vi "Get Boolean Trigger.vi"(7 "Trigger Direction":T1, 8 "error in (no error)":errorcluster, 11 "Item Ref in":T3 format="%.0x") -> (0 "error out":errorcluster, 2 "Boolean Trigger":T2, 3 "Item Ref out":T3 format="%.0x")   [LabVIEW 2012, in "Waveform Data Logger Shared.lvlib"]
uses:
  Waveform Data Logger Shared.lvlib
  <vilib>/NI Veristand/Custom Device API/Custom Device Item Ref.ctl
  Types/Boolean Trigger.ctl
  Types/Trigger Direction.ctl
  Globals/Property Strings.vi
  <vilib>/NI Veristand/Custom Device API/Get Item Property (Double).vi
  <vilib>/NI Veristand/Custom Device API/Get Item Property (U16).vi
  <vilib>/NI VeriStand/Custom Device API/Custom Device API.lvlib
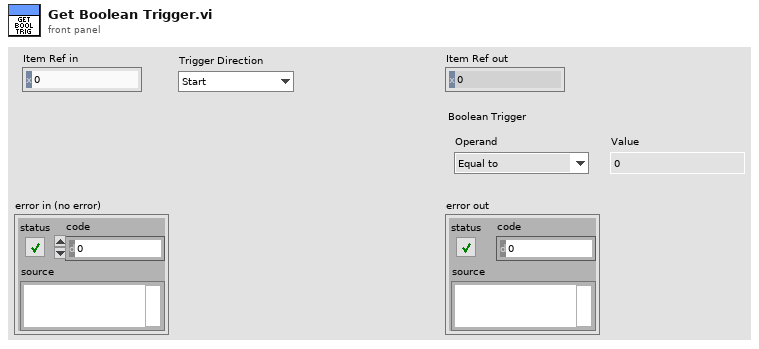
[diagram p1: front panel]
types:
  T1 = typedef "Waveform Data Logger Shared.lvlib/Trigger Direction.ctl" = enum16{"Start", "Stop"}
  T2 = typedef "Waveform Data Logger Shared.lvlib/Boolean Trigger.ctl" = cluster{"Value":dbl, "Operand":enum16{"Equal to", "Not equal to", "Less than", "Less than or equal", "Greater than", "Greater than or equal"}}
  T3 = typedef "Custom Device API.lvlib/Custom Device Item Ref.ctl" = u64
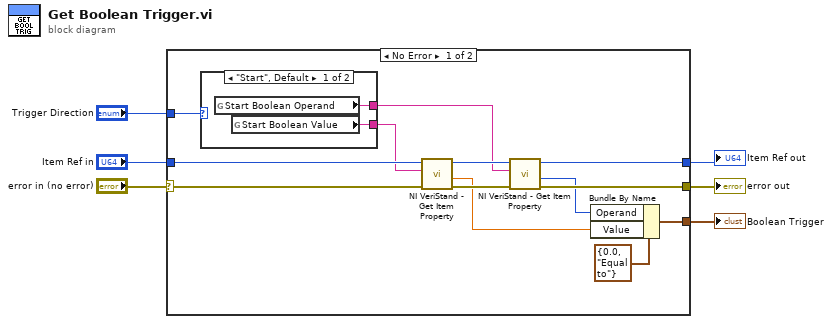
[diagram p0: block diagram]
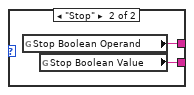
[diagram p2: hidden frame]
diagram:
  n1 = case shown="No Error" "error in (no error)" {
    selector: "error in (no error)" -> [w16 w24]
    tunnel: [w14 w25] -> w6
    tunnel: [w11 w24] -> w5
    tunnel: "Item Ref in" -> [w17 w25]
    tunnel: "Trigger Direction" -> [w19 _]
    tunnel: [w7 _] -> w1
    frame No Error {
      n2 = case shown="\"Start\", Default" w19 {
        tunnel: [w21 w23] -> w10
        tunnel: [w20 w22] -> w15
        frame "Start", Default {
          n3 = global read "Property Strings.vi" "Start Boolean Operand"() -> (w21:string)
          n4 = global read "Property Strings.vi" "Start Boolean Value"() -> (w20:string)
        }
        frame "Stop" {
          n5 = global read "Property Strings.vi" "Stop Boolean Operand"() -> (w23:string)
          n6 = global read "Property Strings.vi" "Stop Boolean Value"() -> (w22:string)
        }
      }
      n7 = call-poly <vilib>:"NI VeriStand - Get Item Property.vi"("error in (no error)"=w16, "Property Name"=w15, "Item Ref in"=w17) -> ("error out"=w12:errorcluster, "Value"=w8:dbl, "Item Ref out"=w13:T3)  [unwired: 1 in, 5 out]
      n8 = call-poly <vilib>:"NI VeriStand - Get Item Property.vi"("error in (no error)"=w12, "Property Name"=w10, "Item Ref in"=w13) -> ("error out"=w11:errorcluster, "Value"=w9:u16, "Item Ref out"=w14:T3)  [unwired: 1 in, 5 out]
      n9 = Bundle By Name(cluster=T2 {"Value"=0.0, "Operand"=enum."Equal to"} ("Boolean Trigger"), "Operand"=w9, "Value"=w8) -> (w7:T2)
    }
    frame Error {
    }
  }
  "Item Ref out" <- w6
  "error out" <- w5
  "Boolean Trigger" <- w1
